vi "RewriteVariantFile.vi"() -> ()   [LabVIEW 2016]
panel:
  in  "output":path=path "output"
  in  "input":path=path "C:/Private/LaserMarkingSystemClear/settings/Variants1.ini"
  out "error out":errorcluster
  out "array type (2D Dbl) 2":string[][](array[string])
  out "array type (2D Dbl)":string[](array[string])
  out "array":string[][](array[string])
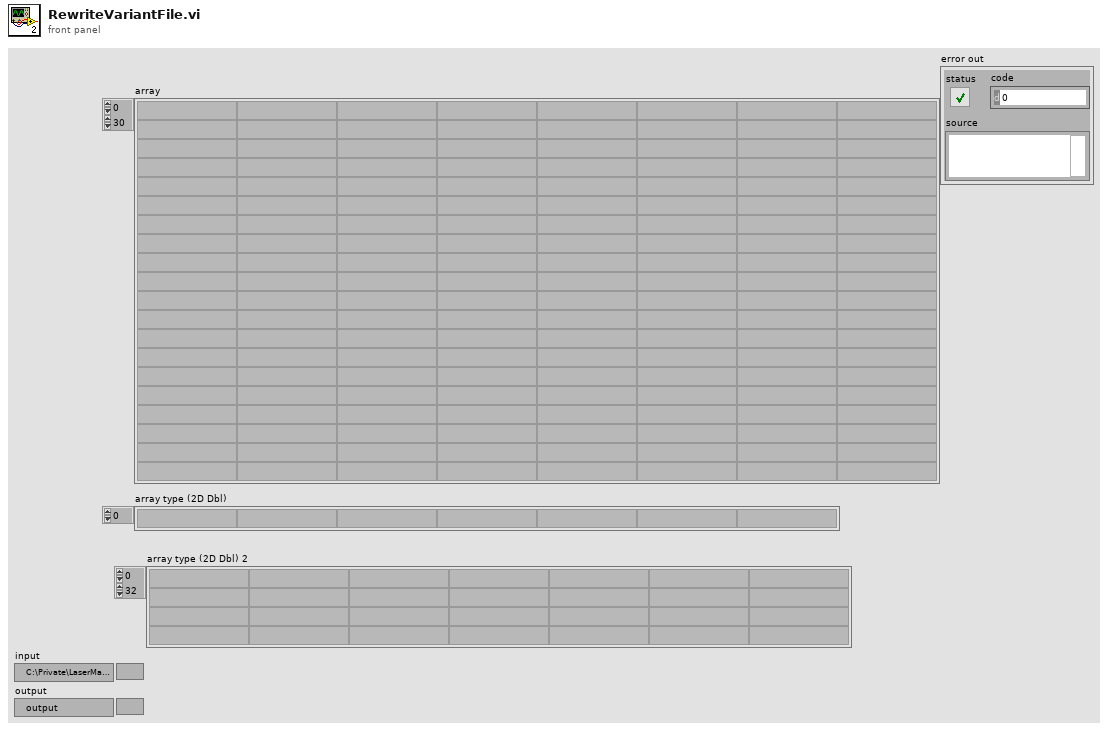
[diagram p1: front panel]
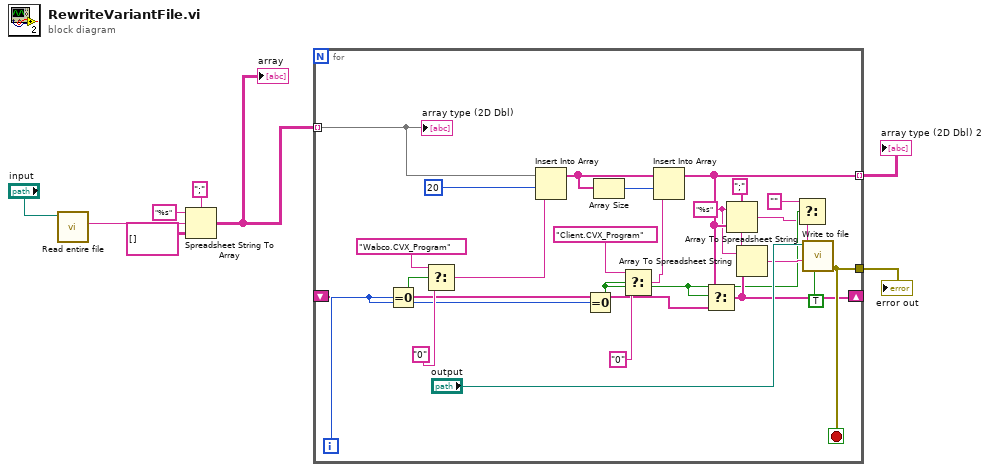
[diagram p0: block diagram]
diagram:
  n1 = call "Read entire file.vi"("file"="input") -> ("contents"=w5:string)  [unwired: 5 in, 1 out]
  n2 = Spreadsheet String To Array(delimiter (Tab)=";", format string="%s", spreadsheet string=w5, array type (2D Dbl)=string[][] []) -> (array=w3:string[][])
  "array" <- w3
  n3 = for {
    tunnel: w3 -> [w33] mode=indexing
    tunnel: [w18] -> w2 mode=indexing
    tunnel: [w20] -> w1
    shift-right: [w14] -> _
    shift-left: _ -> [w17]
    i -> [w19]
    stop <- w20 stop-if-true
    w16 = "%s" ("format string")
    w15 = ";" ("delimiter (Tab)")
    n4 = Equal To 0?(x=w19) -> (x = 0?=w31:bool)
    n5 = Select(t="Wabco.CVX_Program", s=w31, f="0") -> (s? t:f=w23:string)
    n6 = Insert Into Array(array=w33, index=20, new element=w23) -> (w28:string[])
    n7 = Equal To 0?(x=w19) -> (x = 0?=w12:bool)
    n8 = Array Size(array=w28) -> (size(s)=w25:i32)
    n9 = Select(t="Client.CVX_Program", s=w12, f="0") -> (s? t:f=w22:string)
    n10 = Insert Into Array(array=w28, index=w25, new element=w22) -> (w18:string[])
    n11 = Select(t=w18, s=w12, f=w17) -> (s? t:f=w14:string[])
    n12 = Array To Spreadsheet String(delimiter (Tab)=w15, array=w18, 3:w16) -> (spreadsheet string=w11:string)
    n13 = Array To Spreadsheet String(delimiter (Tab)=w15, array=w14, 3:w16) -> (spreadsheet string=w13:string)
    n14 = Select(t="", s=w12, f=w11) -> (s? t:f=w9:string)
    n15 = call "Write to file.vi"("append (F)"=TRUE, "header"=w13, "addition"=w9, "file"="output") -> ("error out"=w20:errorcluster)  [unwired: 7 in]
    "array type (2D Dbl)" <- w33
  }
  "array type (2D Dbl) 2" <- w2
  "error out" <- w1
